vi "Drive and Climb SS Safety 2017.vi"(11 "Drive Actuator In":T1) -> (3 "Drive Actuator Out":T1)   [LabVIEW 2016]
uses:
  Drive Actuator Out 2017.ctl
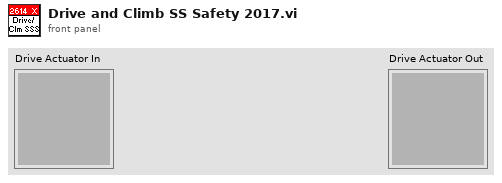
[diagram p1: front panel]
types:
  T1 = typedef "Drive Actuator Out 2017.ctl" = cluster{}
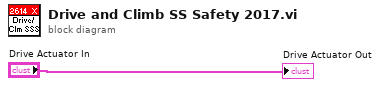
[diagram p0: block diagram]
diagram:
  "Drive Actuator Out" <- "Drive Actuator In"
